vi "Car Wash controller.vi"() -> ()   [LabVIEW 2017]
uses:
  Bundyra/controls/MHL Status.ctl
  Bundyra/controls/MHL UI Data.ctl
  Bundyra/support/Boiler System Globals.vi
  Bundyra/support/Message Queue/Message Queue.lvlib
  Bundyra/Controller/Controller.lvlib
  <vilib>/Utility/error.llb/Error Cluster From Error Code.vi
  <vilib>/ErrorRing/Error Ring.xnode
  Bundyra/support/Message Queue/Message Cluster.ctl
  Bundyra/support/Message Queue/All Message Queues.ctl
  Notifiers.ctl
  Bundyra/Controller/Controller Configuration.ctl
panel:
  in  "Controller Configuration Data":T1
  in  "Notifiers":T2
  in  "Message Queues":T3
  in  "error in":errorcluster
  out "error out":errorcluster
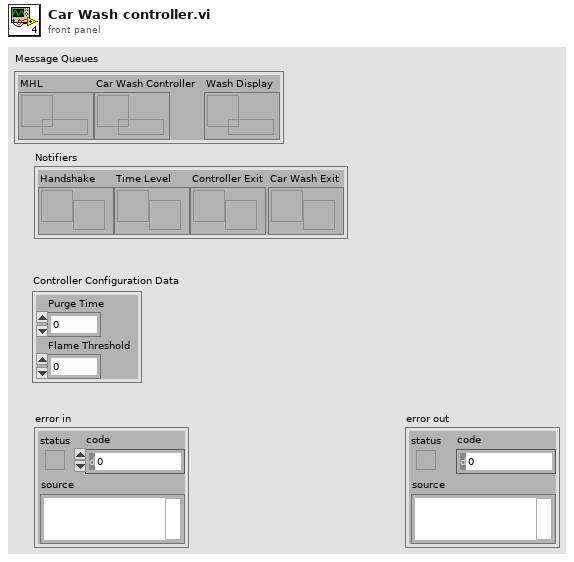
[diagram p1: front panel]
types:
  T1 = typedef "Controller.lvlib/Controller Configuration.ctl" = cluster{"Purge Time":u32, "Flame Threshold":u32}
  T2 = typedef "Notifiers.ctl" = cluster{"Handshake":refnum<notifier>, "Time Level":refnum<notifier>, "Controller Exit":refnum<notifier>, "Car Wash Exit":refnum<notifier>}
  T3 = typedef "Message Queue.lvlib/All Message Queues.ctl" = cluster{"MHL":refnum<queue>, "Car Wash Controller":refnum<queue>, "Wash Display":refnum<queue>}
  T4 = enum16{"open", "replace", "create", "open or create", "replace or create", "replace or create with confirmation"}
  T5 = typedef "MHL Status.ctl" = enum16{"Lockout", "Ready", "Pre-Purge", "Pre-Purge Complete", "Pilot On", "Boiler Running", "Shutdown", "Purge"}
  T6 = typedef "MHL UI Data.ctl" = cluster{"Status":string, "Fuel Control Valve":u32, "Primary Fan":bool, "Pilot Gas Valve":bool, "Pilot":bool, "Forced Draft Fan":bool, "MHL Status":T5}
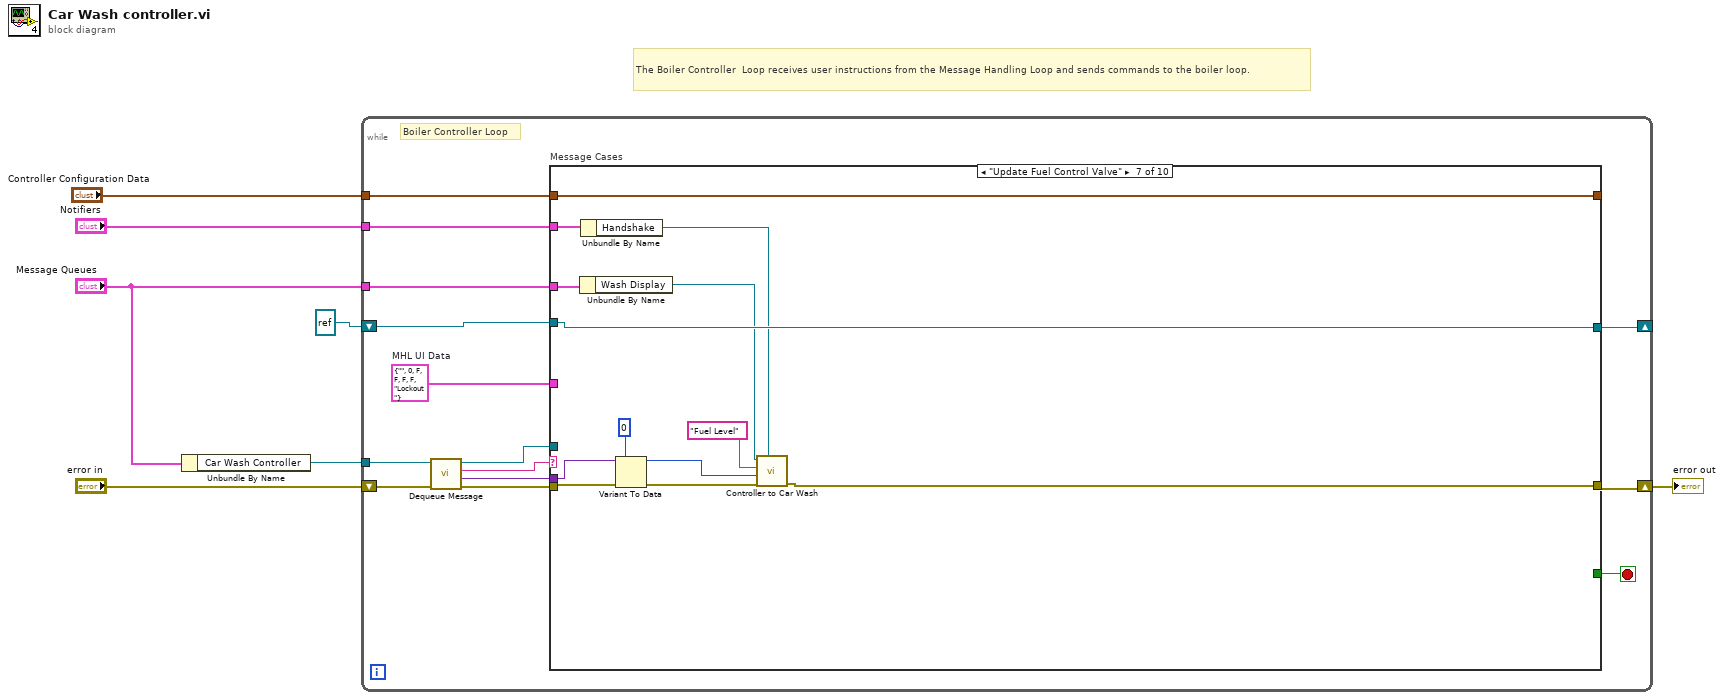
[diagram p0: block diagram]
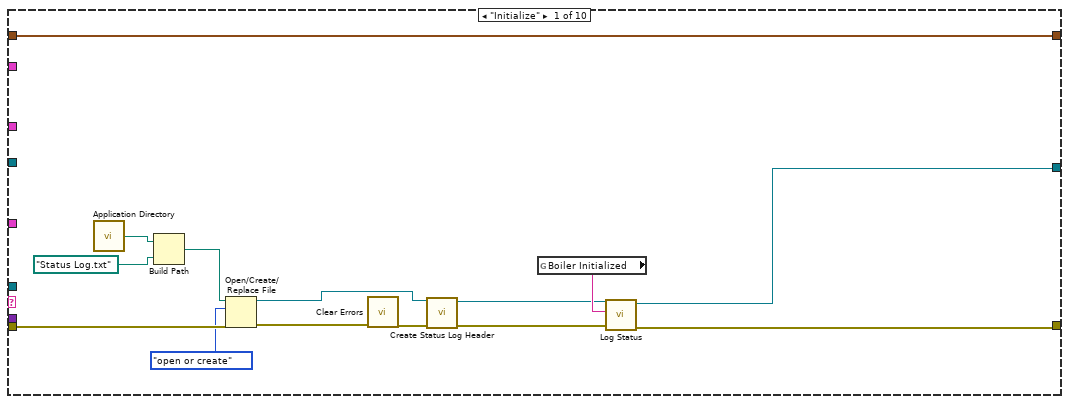
[diagram p2: hidden frame]
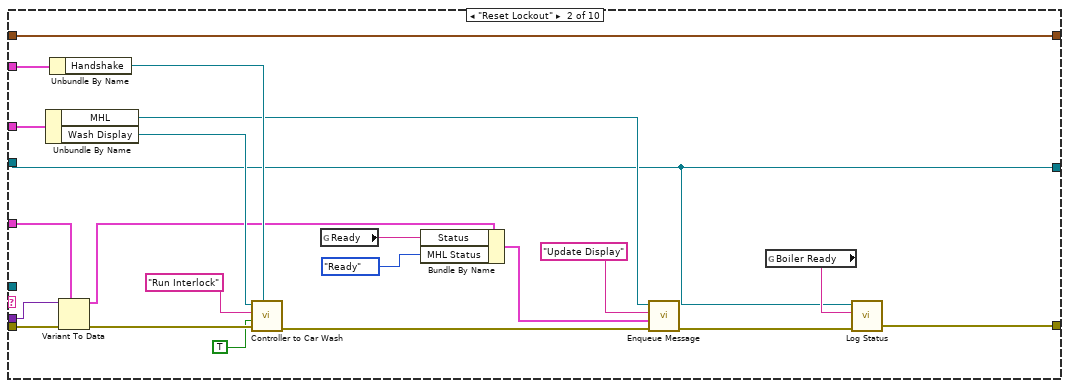
[diagram p3: hidden frame]
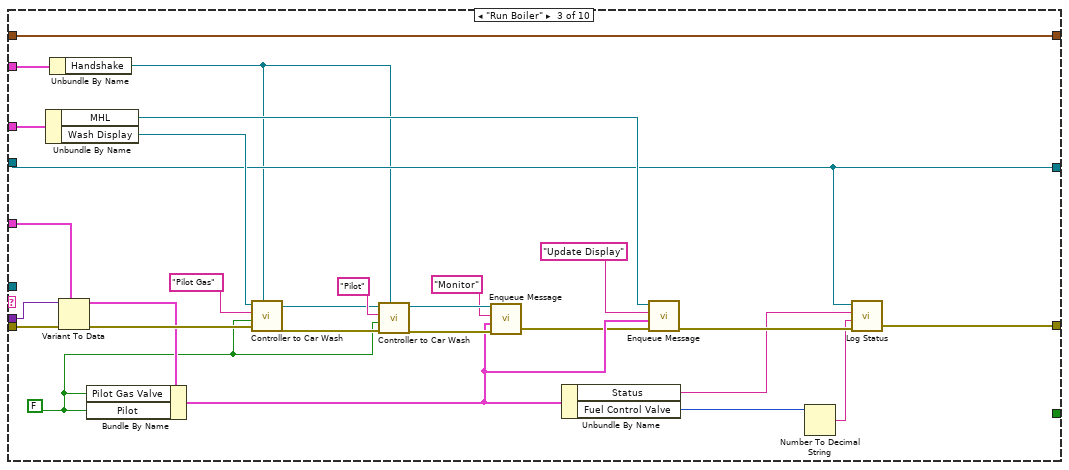
[diagram p4: hidden frame]
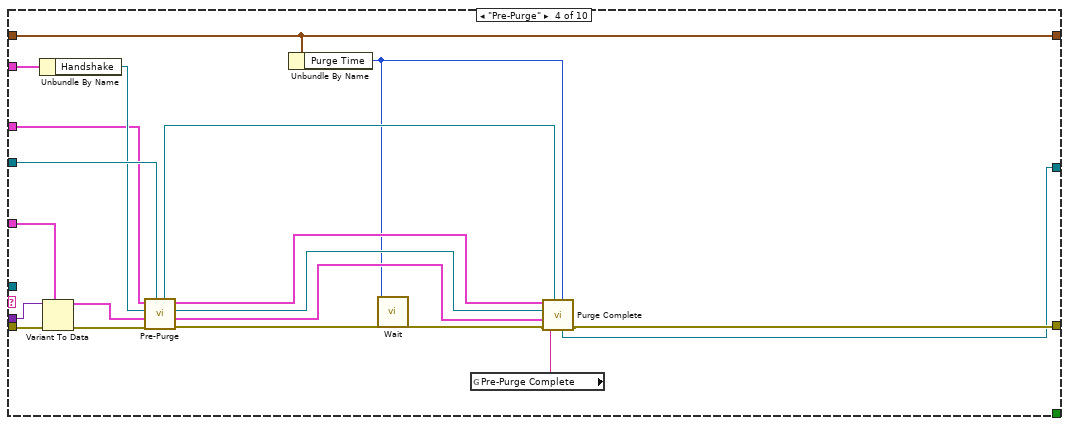
[diagram p5: hidden frame]
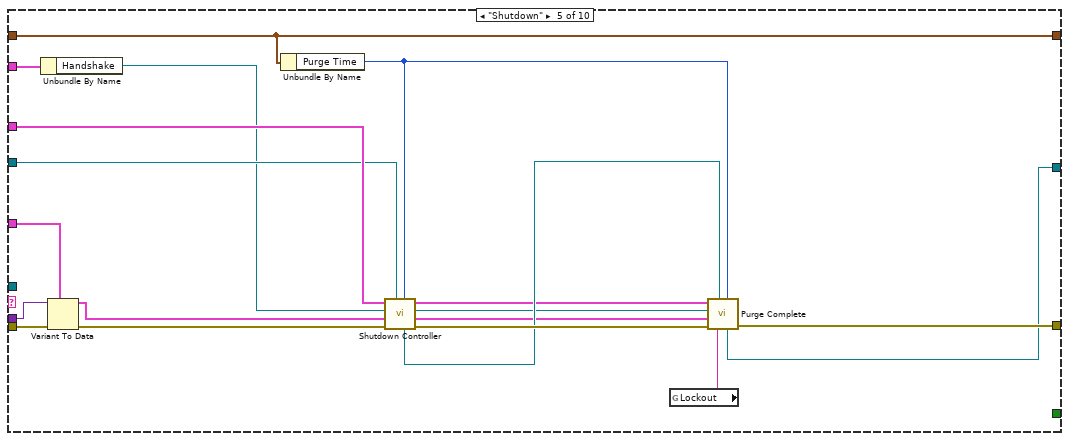
[diagram p6: hidden frame]
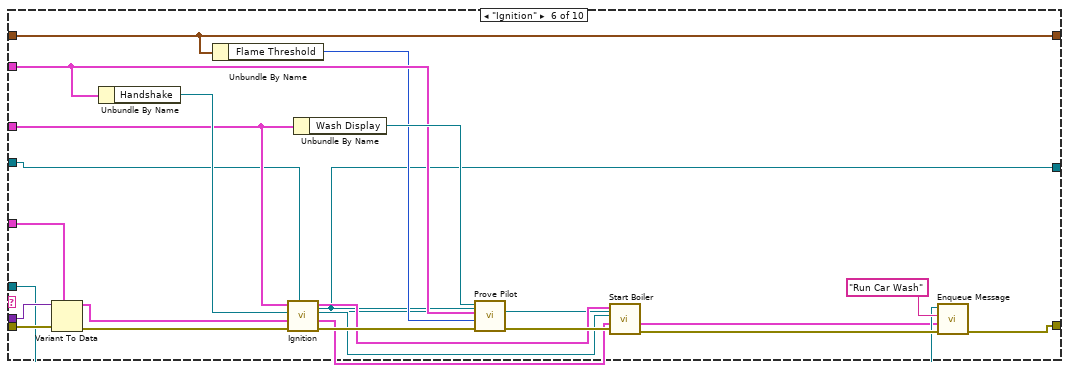
[diagram p7: hidden frame]
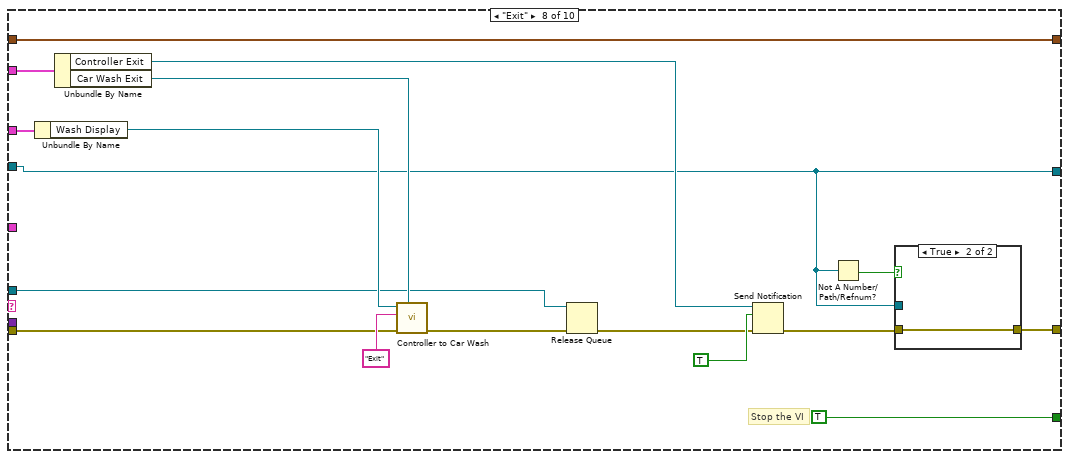
[diagram p8: hidden frame]
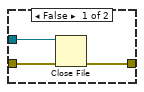
[diagram p9: hidden frame]
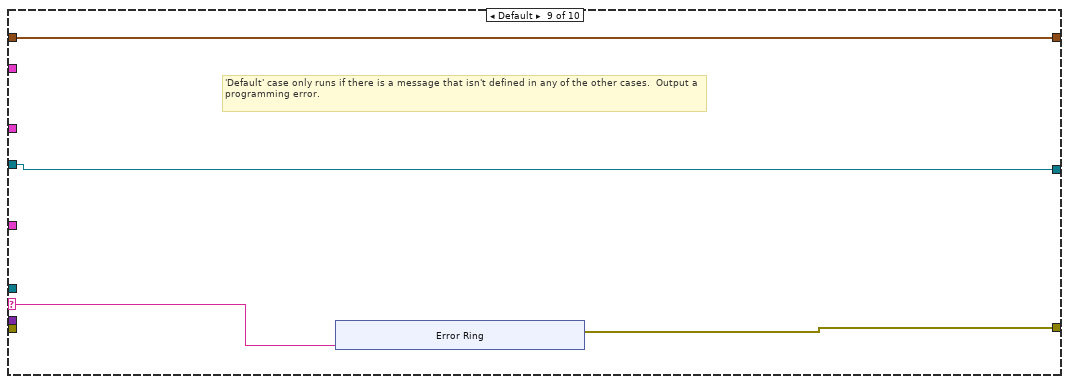
[diagram p10: hidden frame]
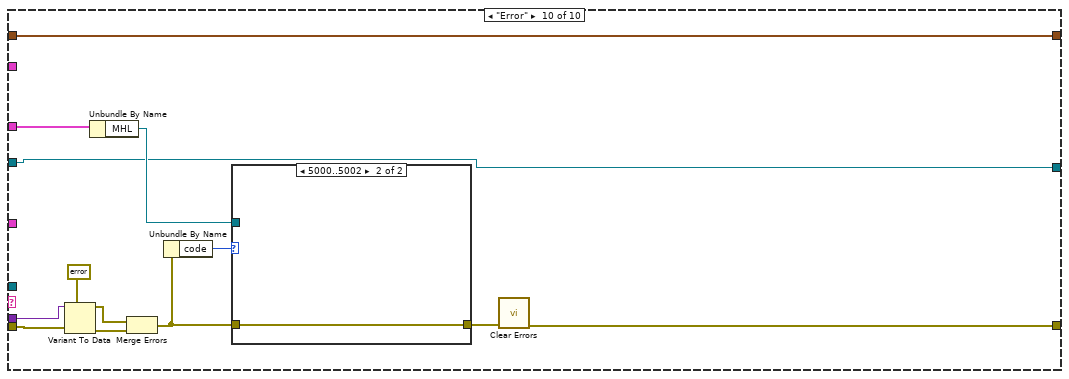
[diagram p11: hidden frame]
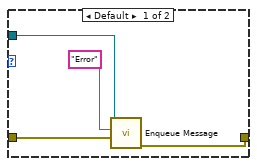
[diagram p12: hidden frame]
diagram:
  # "The Boiler Controller  Loop receives user instructions from the Message Handling Loop and sends commands to the boiler loop."
  n1 = Unbundle By Name("Message Queues") -> ("Car Wash Controller"=w5:refnum<queue>)
  n2 = while {
    tunnel: w5 -> [w15]
    shift-right: [w14] -> w7
    shift-left: "error in" -> [w20]
    tunnel: "Message Queues" -> [w13]
    tunnel: "Notifiers" -> [w12]
    shift-right: [w10] -> _
    shift-left: refnum<file> refnum ("Log File Refnum Out") -> [w11]
    tunnel: "Controller Configuration Data" -> [w8]
    stop <- w21 stop-if-true
    w9 = T6 {"Status"="", "Fuel Control Valve"=0, "Primary Fan"=FALSE, "Pilot Gas Valve"=FALSE, "Pilot"=FALSE, "Forced Draft Fan"=FALSE, "MHL Status"=enum."Lockout"}  # MHL UI Data
    # "Boiler Controller Loop"
    n3 = call "Dequeue Message.vi"("error in (no error)"=w20, "Message Queue"=w15) -> ("error out"=w19:errorcluster, "Message Data"=w17:variant, "Message"=w18:string, "dup Message Queue"=w16:refnum<queue>)  [unwired: 6 in]
    n4 = case "Message Cases" shown="\"Update Fuel Control Valve\"" w18 {
      selector: w18 -> [_ _ _ _ _ _ _ _ w184 _]
      tunnel: w16 -> [_ _ _ _ _ w126 _ w170 _ _]
      tunnel: w19 -> [w33 w55 w83 w101 w124 w146 w158 w169 _ w201]
      tunnel: [w24 w38 w73 w93 w113 w129 w148 w163 w185 w195] -> w14
      tunnel: [_ _ _ _ _ _ _ TRUE _ _] -> w21
      tunnel: w17 -> [_ w54 w82 w97 w123 w131 w155 _ _ w200]
      tunnel: w13 -> [_ w56 w84 w102 w119 w141 w151 w167 _ w205]
      tunnel: w12 -> [_ w57 w85 w105 w120 w138 w152 w166 _ _]
      tunnel: w11 -> [_ w39 w74 w104 w118 w140 w160 w162 w183 w194]
      tunnel: [w23 w39 w74 w86 w106 w132 w160 w162 w183 w194] -> w10
      tunnel: w9 -> [_ w53 w81 w98 w122 w130 _ _ _ _]
      tunnel: w8 -> [w22 w36 w72 w96 w121 w147 w159 w161 w182 w193]
      tunnel: [w22 w36 w72 w96 w121 w147 w159 w161 w182 w193] -> _
      frame "Initialize" {
        n5 = call <vilib>:"Application Directory.vi"() -> ("Application Directory"=w34:path)
        n6 = Build Path(base path=w34, name or relative path=path "Status Log.txt") -> (appended path=w31:path)
        n7 = Open/Create/Replace File(file path (use dialog)=w31, error in=w33, operation (0:open)=T4."open or create") -> (refnum out=w26:refnum<file>, error out=w30:errorcluster)  [unwired: 3 in, 1 out]
        n8 = call <vilib>:"Clear Errors.vi"("error in (no error)"=w30) -> ("error out"=w29:errorcluster)  [unwired: 5 in, 1 out]
        n9 = call "Create Status Log Header.vi"("error in"=w29, "Log File Refnum in"=w26) -> ("error out"=w28:errorcluster, "Log File Refnum out"=w25:refnum<file>)  [unwired: 8 in]
        n10 = global read "Boiler System Globals.vi" "Boiler Initialized"() -> (w27:string)
        n11 = call "Log Status.vi"("error in"=w28, "Event String"=w27, "Log File Refnum In"=w25) -> ("error out"=w24:errorcluster, "Log File Refnum Out"=w23:refnum<file>)  [unwired: 7 in]
      }
      frame "Reset Lockout" {
        n12 = Unbundle By Name(w56) -> ("MHL"=w43:refnum<queue>, "Wash Display"=w50:refnum<queue>)
        n13 = Unbundle By Name(w57) -> ("Handshake"=w49:refnum<notifier>)
        n14 = Variant To Data(error in=w55, type=w53, Variant=w54) -> (data=w46:T6, error out=w51:errorcluster)
        n15 = call "Controller to Car Wash.vi"("Notifier"=w49, "error in"=w51, "Message Data"=TRUE, "Message"="Run Interlock", "Car wash Queue in"=w50) -> ("error out"=w42:errorcluster)  [unwired: 4 in, 2 out]
        n16 = global read "Boiler System Globals.vi" "Ready"() -> (w52:string)
        n17 = Bundle By Name(cluster=w46, "Status"=w52, "MHL Status"=MHL_Status."Ready") -> (w45:T6)
        n18 = call "Enqueue Message.vi"("error in (no error)"=w42, "Message Data"=w45, "Message"="Update Display", "Message Queue"=w43) -> ("error out"=w41:errorcluster)  [unwired: 6 in, 1 out]
        n19 = global read "Boiler System Globals.vi" "Boiler Ready"() -> (w40:string)
        n20 = call "Log Status.vi"("error in"=w41, "Event String"=w40, "Log File Refnum In"=w39) -> ("error out"=w38:errorcluster)  [unwired: 7 in, 1 out]
      }
      frame "Run Boiler" {
        w67 = FALSE
        n21 = Unbundle By Name(w84) -> ("MHL"=w76:refnum<queue>, "Wash Display"=w79:refnum<queue>)
        n22 = Unbundle By Name(w85) -> ("Handshake"=w58:refnum<notifier>)
        n23 = Variant To Data(error in=w83, type=w81, Variant=w82) -> (data=w71:T6, error out=w80:errorcluster)
        n24 = Bundle By Name(cluster=w71, "Pilot Gas Valve"=w67, "Pilot"=w67) -> (w63:T6)
        n25 = call "Controller to Car Wash.vi"("Notifier"=w58, "error in"=w80, "Message Data"=w67, "Message"="Pilot Gas", "Car wash Queue in"=w79) -> ("error out"=w68:errorcluster, "Queue out"=w69:refnum<queue>)  [unwired: 4 in, 1 out]
        n26 = call "Controller to Car Wash.vi"("Notifier"=w58, "error in"=w68, "Message Data"=w67, "Message"="Pilot", "Car wash Queue in"=w69) -> ("error out"=w65:errorcluster, "Queue out"=w66:refnum<queue>)  [unwired: 4 in, 1 out]
        n27 = call "Enqueue Message.vi"("error in (no error)"=w65, "Message Data"=w63, "Message"="Monitor", "Message Queue"=w66) -> ("error out"=w62:errorcluster)  [unwired: 6 in, 1 out]
        n28 = Unbundle By Name(w63) -> ("Status"=w61:string, "Fuel Control Valve"=w60:u32)
        n29 = call "Enqueue Message.vi"("error in (no error)"=w62, "Message Data"=w63, "Message"="Update Display", "Message Queue"=w76) -> ("error out"=w75:errorcluster)  [unwired: 6 in, 1 out]
        n30 = Number To Decimal String(number=w60) -> (decimal integer string=w59:string)  [unwired: 1 in]
        n31 = call "Log Status.vi"("error in"=w75, "Event Data String (-)"=w59, "Event String"=w61, "Log File Refnum In"=w74) -> ("error out"=w73:errorcluster)  [unwired: 6 in, 1 out]
      }
      frame "Pre-Purge" {
        n32 = Unbundle By Name(w105) -> ("Handshake"=w103:refnum<notifier>)
        n33 = Variant To Data(error in=w101, type=w98, Variant=w97) -> (data=w99:T6, error out=w100:errorcluster)
        n34 = call "Pre-Purge.vi"("Log File Refnum in"=w104, "error in"=w100, "UI Data in"=w99, "Handshake Notifier in"=w103, "Message Queues in"=w102) -> ("error out"=w95:errorcluster, "UI Data out"=w88:T6, "Handshake Notifier out"=w89:refnum<notifier>, "Message Queues out"=w90:T3, "Log File Refnum out"=w91:refnum<file>)  [unwired: 2 in]
        n35 = Unbundle By Name(w96) -> ("Purge Time"=w87:u32)
        n36 = call "Wait.vi"("error in"=w95, "Purge Time (s)"=w87) -> ("error out"=w94:errorcluster)  [unwired: 9 in]
        n37 = global read "Boiler System Globals.vi" "Pre-Purge Complete"() -> (w92:string)
        n38 = call "Purge Complete.vi"("Purge Time"=w87, "Status"=w92, "Log File Refnum in"=w91, "error in"=w94, "UI Data in"=w88, "Handshake Notifier in"=w89, "Message Queues in"=w90) -> ("error out"=w93:errorcluster, "Log File Refnum out"=w86:refnum<file>)  [unwired: 3 out]
      }
      frame "Shutdown" {
        n39 = Unbundle By Name(w120) -> ("Handshake"=w117:refnum<notifier>)
        n40 = Variant To Data(error in=w124, type=w122, Variant=w123) -> (data=w116:T6, error out=w115:errorcluster)
        n41 = Unbundle By Name(w121) -> ("Purge Time"=w111:u32)
        n42 = call "Shutdown Controller.vi"("Purge Time"=w111, "Log File Refnum in"=w118, "error in"=w115, "UI Data in"=w116, "Handshake Notifier in"=w117, "Message Queues in"=w119) -> ("error out"=w114:errorcluster, "UI Data out"=w108:T6, "Handshake Notifier out"=w109:refnum<notifier>, "Message Queues out"=w110:T3, "Log File Refnum out"=w112:refnum<file>)  [unwired: 1 in]
        n43 = global read "Boiler System Globals.vi" "Lockout"() -> (w107:string)
        n44 = call "Purge Complete.vi"("Purge Time"=w111, "Status"=w107, "Log File Refnum in"=w112, "error in"=w114, "UI Data in"=w108, "Handshake Notifier in"=w109, "Message Queues in"=w110) -> ("error out"=w113:errorcluster, "Log File Refnum out"=w106:refnum<file>)  [unwired: 3 out]
      }
      frame "Ignition" {
        n45 = Variant To Data(error in=w146, type=w130, Variant=w131) -> (data=w143:T6, error out=w145:errorcluster)
        n46 = Unbundle By Name(w138) -> ("Handshake"=w142:refnum<notifier>)
        n47 = Unbundle By Name(w147) -> ("Flame Threshold"=w137:u32)
        n48 = call "Ignition.vi"("Log File Refnum in"=w140, "error in"=w145, "UI Data in"=w143, "Handshake Notifier in"=w142, "Message Queues in"=w141) -> ("error out"=w144:errorcluster, "UI Data out"=w133:T6, "Handshake Notifier out"=w134:refnum<notifier>, "Message Queues out"=w135:T3, "Log File Refnum out"=w132:refnum<file>)  [unwired: 2 in]
        n49 = Unbundle By Name(w141) -> ("Wash Display"=w139:refnum<queue>)
        n50 = call "Prove Pilot.vi"("Log File Refnum in"=w132, "error in"=w144, "Flame Threshold"=w137, "Notifiers in"=w138, "Boiler Queue in"=w139) -> ("error out"=w136:errorcluster)  [unwired: 3 in, 3 out]
        n51 = call "Start Boiler.vi"("Log File Refnum in"=w132, "error in"=w136, "UI Data in"=w133, "Handshake Notifier in"=w134, "Message Queues in"=w135) -> ("error out"=w128:errorcluster, "UI Data out"=w125:T6)  [unwired: 2 in, 3 out]
        n52 = call "Enqueue Message.vi"("error in (no error)"=w128, "Message Data"=w125, "Message"="Run Car Wash", "Message Queue"=w126) -> ("error out"=w129:errorcluster)  [unwired: 6 in, 1 out]
      }
      frame "Update Fuel Control Valve" {
        n53 = Unbundle By Name(w151) -> ("Wash Display"=w149:refnum<queue>)
        n54 = Unbundle By Name(w152) -> ("Handshake"=w150:refnum<notifier>)
        n55 = Variant To Data(error in=w158, type=u32 0, Variant=w155) -> (data=w153:u32, error out=w157:errorcluster)
        n56 = call "Controller to Car Wash.vi"("Notifier"=w150, "error in"=w157, "Message Data"=w153, "Message"="Fuel Level", "Car wash Queue in"=w149) -> ("error out"=w148:errorcluster)  [unwired: 4 in, 2 out]
      }
      frame "Exit" {
        # "Stop the VI"
        n57 = Unbundle By Name(w167) -> ("Wash Display"=w171:refnum<queue>)
        n58 = Unbundle By Name(w166) -> ("Controller Exit"=w172:refnum<notifier>, "Car Wash Exit"=w174:refnum<notifier>)
        n59 = call "Controller to Car Wash.vi"("Notifier"=w174, "error in"=w169, "Message"="Exit", "Car wash Queue in"=w171) -> ("error out"=w177:errorcluster)  [unwired: 5 in, 2 out]
        n60 = Release Queue(queue=w170, error in (no error)=w177) -> (error out=w173:errorcluster)  [unwired: 1 in, 2 out]
        n61 = Send Notification(notification=TRUE, notifier=w172, error in (no error)=w173) -> (error out=w164:errorcluster)  [unwired: 1 out]
        n62 = Not A Number/Path/Refnum?(number/path/refnum=w162) -> (NaN/Path/Refnum?=w165:bool)
        n63 = case shown="True" w165 {
          tunnel: w164 -> [w180 w181]
          tunnel: [w179 w181] -> w163
          tunnel: w162 -> [w178 _]
          frame False {
            n64 = Close File(refnum=w178, error in=w180) -> (error out=w179:errorcluster)  [unwired: 1 out]
          }
          frame True {
          }
        }
      }
      frame Default {
        # "'Default' case only runs if there is a message that isn't defined in any of the other cases.  Output a programming error."
        n65 = xnode "Error Ring"("parameter 0"=w184) -> ("error out"=w185:errorcluster)
      }
      frame "Error" {
        n66 = Variant To Data(error in=w201, type=errorcluster {"status"=FALSE, "code"=0, "source"=""} ("error out"), Variant=w200) -> (data=w202:errorcluster, error out=w203:errorcluster)
        n67 = Unbundle By Name(w205) -> ("MHL"=w197:refnum<queue>)
        n68 = Merge Errors(w202, w203) -> (w198:errorcluster)
        n69 = Unbundle By Name(w198) -> ("code"=w199:i32)
        n70 = case shown="5000..5002" w199 {
          tunnel: w198 -> [w207 w210]
          tunnel: w197 -> [w208 _]
          tunnel: [w206 w210] -> w196
          frame Default {
            n71 = call "Enqueue Message.vi"("Message Data"=w207, "Message"="Error", "Message Queue"=w208) -> ("error out"=w206:errorcluster)  [unwired: 7 in, 1 out]
          }
          frame 5000..5002 {
          }
        }
        n72 = call <vilib>:"Clear Errors.vi"("error in (no error)"=w196) -> ("error out"=w195:errorcluster)  [unwired: 5 in, 1 out]
      }
    }
  }
  "error out" <- w7
